vi "Test Setup Error Dummy.vi"(8 "error in (no error)":errorcluster, 11 "Setup Error Test Dummy in":refnum<class "Setup Error Test Dummy.lvclass">) -> (0 "error out":errorcluster, 3 "Setup Error Test Dummy out":refnum<class "Setup Error Test Dummy.lvclass">)   [LabVIEW 2020, in "Setup Error Test Dummy.lvclass"]
uses:
  Setup Error Test Dummy.lvclass
  C:/git/astemes-lunit/source/LUnit Test Case.lvclass
  source/LUnit Test Case.lvclass/LUnit Test Case.ctl
  source/Core/LUnit Test Case/Private/Append Pass Result.vi
  source/Core/LUnit Test Case/Private/Run In UI.vi
  <vilib>/Utility/error.llb/Clear Errors.vi
  source/LUnit Test Case.lvclass
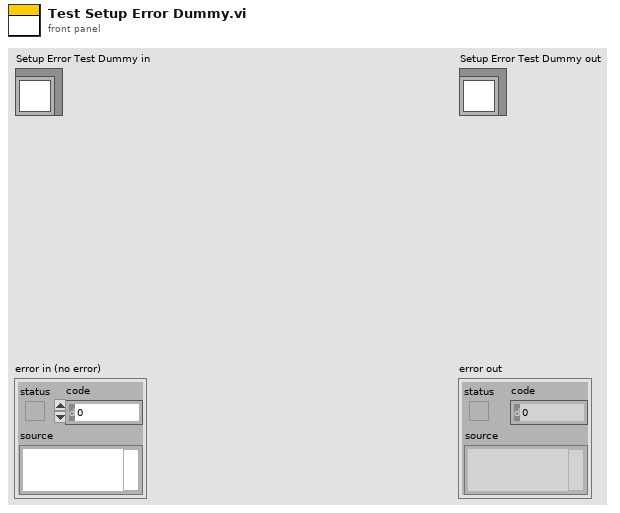
[diagram p1: front panel]
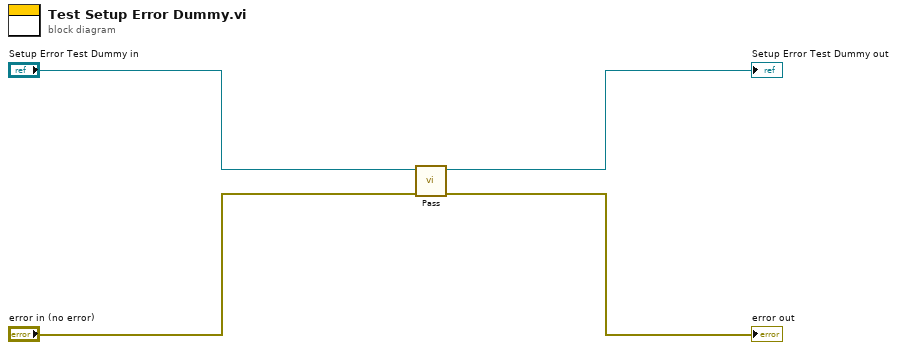
[diagram p0: block diagram]
diagram:
  n1 = call "Pass.vi"("error in (no error)"="error in (no error)", "LUnit Test Case In"="Setup Error Test Dummy in") -> ("error out"=→"error out":errorcluster, "LUnit Test Case Out"=→"Setup Error Test Dummy out":refnum<class "Setup Error Test Dummy.lvclass">)  [unwired: 8 in]
